vi "Device Index by Name.vi"(8 "error in (no error)":errorcluster, 10 "Device Name":string, 11 "HAL Editor in":refnum<class "HAL Editor.lvclass">) -> (0 "error out":errorcluster, 2 "Device Index":i32, 3 "HAL Editor out":refnum<class "HAL Editor.lvclass">)   [LabVIEW 2012, in "HAL Config.lvlib" / "HAL Editor.lvclass"]
uses:
  HAL Editor.lvclass
  build/ppl/lv-hal.lvlibp/Device/Device.lvclass
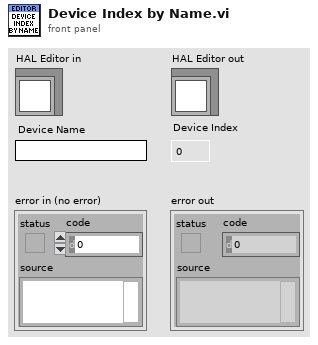
[diagram p1: front panel]
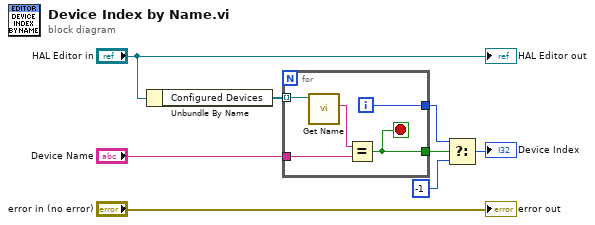
[diagram p0: block diagram]
diagram:
  n1 = Unbundle By Name("HAL Editor in") -> ("Configured Devices"=w6:refnum<class "Device.lvclass">[])
  n2 = for {
    tunnel: w6 -> [w13] mode=indexing
    tunnel: "Device Name" -> [w11]
    tunnel: [w10] -> w4
    tunnel: [w9] -> w3
    i -> [w9]
    stop <- w10 stop-if-true
    n3 = call "Get Name.vi"("Device in"=w13) -> ("Name"=w12:string)  [unwired: 8 in, 2 out]
    n4 = Equal?(x=w12, y=w11) -> (x = y?=w10:bool)
  }
  n5 = Select(t=w3, s=w4, f=-1) -> (s? t:f=→"Device Index":i32)
  "error out" <- "error in (no error)"
  "HAL Editor out" <- "HAL Editor in"
